vi "Configure Measurement (Demodulation - ASK or FSK).vi"(0 "VISA resource name":refnum<visa-resource-name>, 1 "Reference Filter (0: RNyquist)":i32(ring) items=["RNyquist", "Nyquist", "Gaussian", "None"], 3 "Symbol Rate (100 Symbols per second)":dbl=100.0, 5 "Filter Alpha/Bbt (0.2)":dbl=0.2, 9 "Measurement Filter (0: None)":i32(ring) items=["None", "RNyquist", "Nyquist", "Gaussian"], 11 "error in (no error)":errorcluster, 12 "Symbol Filter (2)":dbl=2.0) -> (4 "VISA resource name out":refnum<visa-resource-name>, 15 "error out":errorcluster)   [LabVIEW 2022 SP3, in "Agilent N934X Series.lvlib"]
doc: "Configures the general setting for ASK or FSK demodulation of Demodulation Option.\n\nNote:\nThis VI is only applicable for N9321C, N9322C, N9323C, N9324C models"
uses:
  <instrlib>/Agilent N934X Series/Agilent N934X Series.lvlib
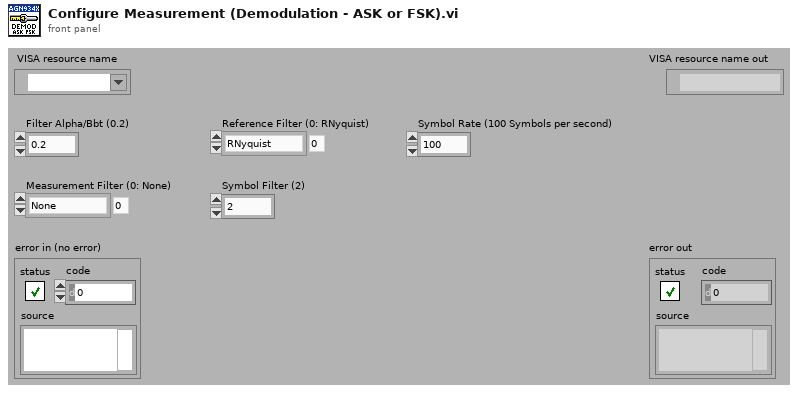
[diagram p1: front panel]
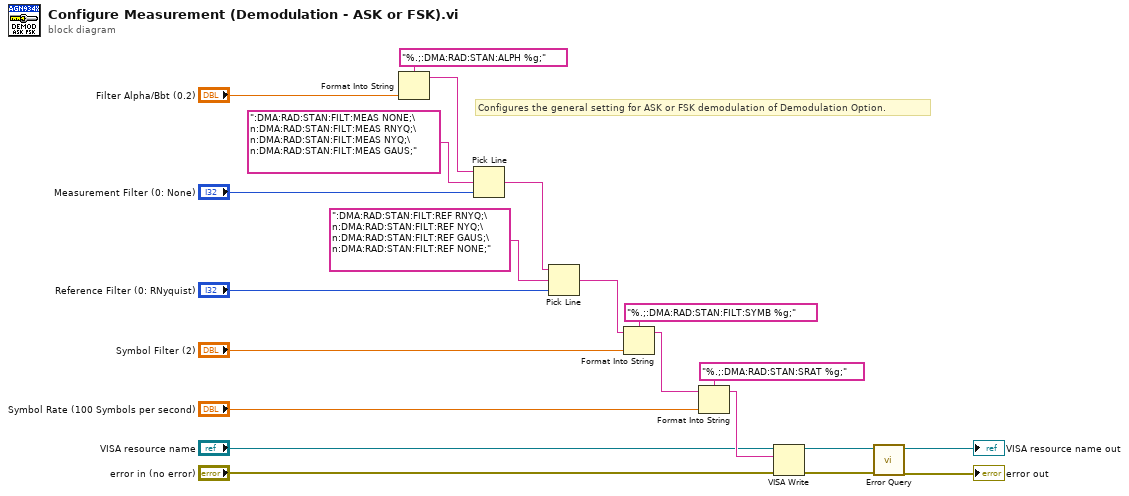
[diagram p0: block diagram]
diagram:
  # "Configures the general setting for ASK or FSK demodulation of Demodulation Option."
  n1 = Format Into String(format string="%.;:DMA:RAD:STAN:ALPH %g;", "Filter Alpha/Bbt (0.2)") -> (resulting string=w17:string)  [unwired: 2 in, 1 out]
  n2 = Pick Line(string ("")=w17, multi-line string=":DMA:RAD:STAN:FILT:MEAS NONE;\n:DMA:RAD:STAN:FILT:MEAS RNYQ;\n:DMA:RAD:STAN:FILT:MEAS NYQ;\n:DMA:RAD:STAN:FILT:MEAS GAUS;", line index="Measurement Filter (0: None)") -> (output string=w14:string)
  n3 = Pick Line(string ("")=w14, multi-line string=":DMA:RAD:STAN:FILT:REF RNYQ;\n:DMA:RAD:STAN:FILT:REF NYQ;\n:DMA:RAD:STAN:FILT:REF GAUS;\n:DMA:RAD:STAN:FILT:REF NONE;", line index="Reference Filter (0: RNyquist)") -> (output string=w13:string)
  n4 = Format Into String(format string="%.;:DMA:RAD:STAN:FILT:SYMB %g;", initial string=w13, "Symbol Filter (2)") -> (resulting string=w10:string)  [unwired: 1 in, 1 out]
  n5 = Format Into String(format string="%.;:DMA:RAD:STAN:SRAT %g;", initial string=w10, "Symbol Rate (100 Symbols per second)") -> (resulting string=w7:string)  [unwired: 1 in, 1 out]
  n6 = VISA Write(VISA resource name="VISA resource name", write buffer=w7, error in (no error)="error in (no error)") -> (VISA resource name out=w4:refnum<visa-resource-name>, error out=w3:errorcluster)  [unwired: 1 out]
  n7 = call <instrlib>:"Error Query.vi"("error in (no error)"=w3, "VISA resource name"=w4) -> ("error out"=→"error out":errorcluster, "VISA resource name out"=→"VISA resource name out":refnum<visa-resource-name>)  [unwired: 6 in, 2 out]
